vi "Difference.vi"(8 "error in":errorcluster, 10 "Time":variant, 11 "Time Stamp in":refnum<class "Time Stamp.lvclass">) -> (0 "error out":errorcluster, 2 "Difference":dbl format="%#_g s", 3 "Time Stamp out":refnum<class "Time Stamp.lvclass">)   [LabVIEW 2024, in "HAL.lvlib" / "Time Stamp.lvclass"]
uses:
  Time Stamp.lvclass
  Time Stamp.lvclass/Time Stamp.ctl
  <vilib>/Utility/Data Type/NI_Data Type.lvlib
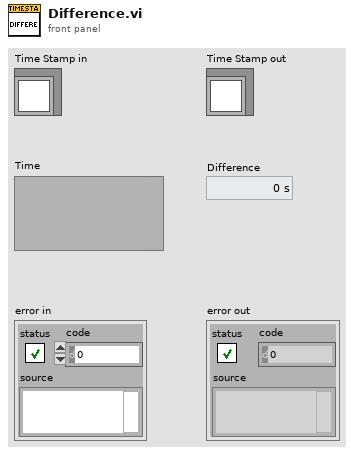
[diagram p1: front panel]
types:
  T1 = typedef "NI_Data Type.lvlib/Data Type.ctl" = enum8{"Invalid Type", "Void", "I8", "I16", "I32", "I64", "U8", "U16", "U32", "U64", "Single Float", "Double Float", "Extended Float", "Single Complex", "Double Complex", "Extended Complex", "Enum U8", "Enum U16", "Enum U32", "Enum U64", "Single Float With Unit", "Double Float With Unit", "Extended Float With Unit", "Single Complex with Unit", "Double Complex with Unit", "Extended Complex with Unit", "Boolean", "String", "Path", "Picture", "Tag", "Array", "Cluster", "Variant", "LV Variant", "Waveform", "Timestamp", "Digital Waveform", "Digital Data", "ExpressData", "Refnum", "External Data", "VI", "Poly VI", "LabVIEW Class Instance", "Fixed Point", "Set Collection", "Map Collection"}
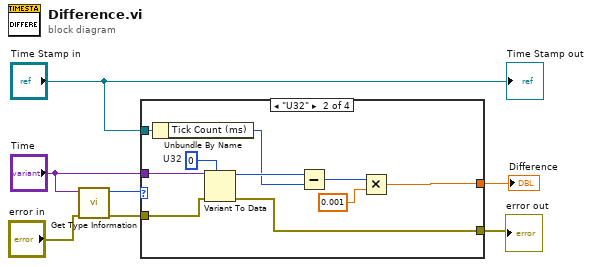
[diagram p0: block diagram]
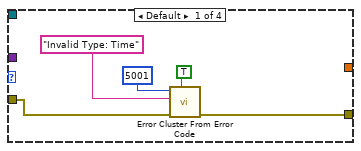
[diagram p2: hidden frame]
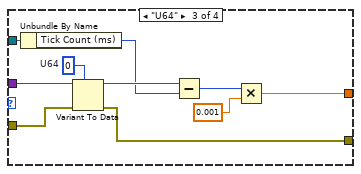
[diagram p3: hidden frame]
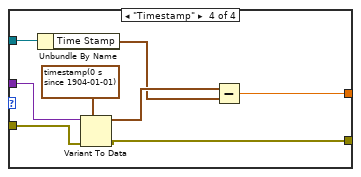
[diagram p4: hidden frame]
diagram:
  n1 = call <vilib>:"Get Type Information.vi"("error in (no error)"="error in", "variant"="Time") -> ("error out"=w4:errorcluster, "type"=w6:T1)  [unwired: 5 in, 3 out]
  n2 = case shown="\"U32\"" w6 {
    tunnel: "Time" -> [_ w22 w26 w39]
    tunnel: w4 -> [w12 w21 w27 w38]
    tunnel: "Time Stamp in" -> [_ w19 w23 w40]
    tunnel: [_ w14 w24 w33] -> w2
    tunnel: [w11 w13 w25 w34] -> w1
    frame Default {
      n3 = call <vilib>:"Error Cluster From Error Code.vi"("show call chain? (False)"=TRUE, "error in (no error)"=w12, "error message (\"\")"="Invalid Type: Time" ("error message (\"\")"), "error code (0)"=5001) -> ("error out"=w11:errorcluster)  [unwired: 5 in]
    }
    frame "U32" {
      w20 = u32 0  # U32
      n4 = Unbundle By Name(w19) -> ("Tick Count (ms)"=w17:u64)
      n5 = Variant To Data(error in=w21, type=w20, Variant=w22) -> (data=w18:u32, error out=w13:errorcluster)
      n6 = Subtract(x=w18, y=w17) -> (x-y=w16:u64)
      n7 = Multiply(x=w16, y=0.001) -> (x*y=w14:dbl)
    }
    frame "U64" {
      w32 = u64 0  # U64
      n8 = Unbundle By Name(w23) -> ("Tick Count (ms)"=w30:u64)
      n9 = Variant To Data(error in=w27, type=w32, Variant=w26) -> (data=w31:u64, error out=w25:errorcluster)
      n10 = Subtract(x=w31, y=w30) -> (x-y=w29:u64)
      n11 = Multiply(x=w29, y=0.001) -> (x*y=w24:dbl)
    }
    frame "Timestamp" {
      n12 = Unbundle By Name(w40) -> ("Time Stamp"=w35:timestamp)
      n13 = Variant To Data(error in=w38, type=timestamp(0 s since 1904-01-01) ("Time Stamp"), Variant=w39) -> (data=w36:timestamp, error out=w34:errorcluster)
      n14 = Subtract(x=w36, y=w35) -> (x-y=w33:dbl)
    }
  }
  "error out" <- w1
  "Difference" <- w2
  "Time Stamp out" <- "Time Stamp in"
